vi "runtest Run Single Test.vi"(6 "TestStation IP (\"\")":string, 7 "Fields In":T1[](array[typedef]), 8 "error in (no error)":errorcluster, 9 "Test Execution Settings":T4={"Quick Mode (T)"=FALSE, "Seq Count"=0, "Step Info"="", "Instruments on Station"=[], "LANGUAGE"="English", "Files Found?"=FALSE, "Step Number"=1} {"Step Number" min=1 step=1}, 10 "Test Configuration (\"\")":string, 11 "Test_ID (\"\")":string) -> (0 "error out":errorcluster, 3 "Fields Out":T1[](array[typedef]), 5 "Test Output":T6)   [LabVIEW 2011]
uses:
  tests/Test Output.ctl
  tests/Test Execution Settings.ctl
  server/database/Stations/Instruments/Instrument Record.ctl
  server/database/Fields/Field Record.ctl
  server/database/Fields/Field DataTypes.ctl
  server/database/Fields/Field NextItem.ctl
  server/database/Fields/Field System Fields.ctl
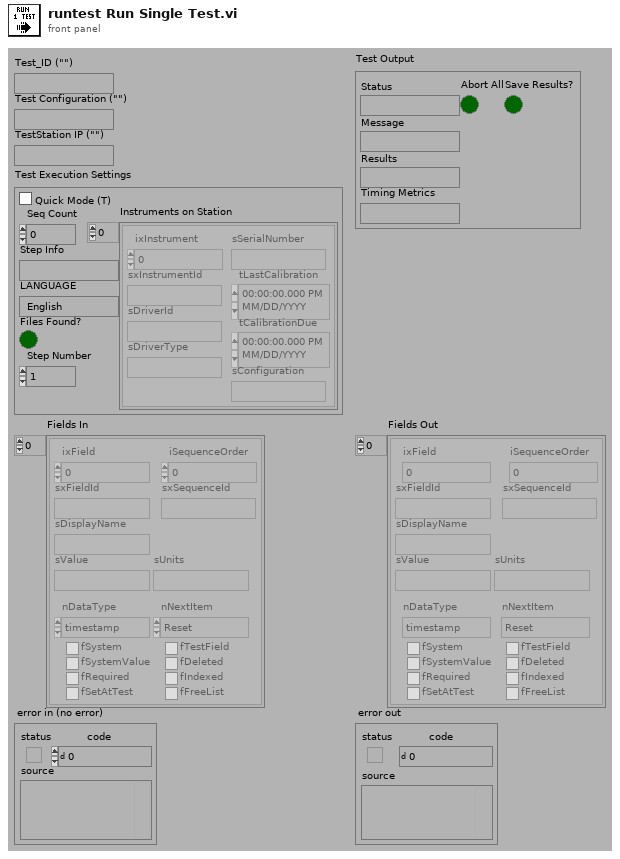
[diagram p1: front panel]
types:
  T1 = typedef "Field Record.ctl" = cluster{"ixField":i32, "iSequenceOrder":i32, "sxFieldId":string, "sxSequenceId":string, "sDisplayName":string, "sValue":string, "sUnits":string, "nDataType":T2, "nNextItem":T3, "fSystem":bool, "fSystemValue":bool, "fRequired":bool, "fSetAtTest":bool, "fTestField":bool, "fDeleted":bool, "fIndexed":bool, "fFreeList":bool}
  T2 = typedef "Field DataTypes.ctl" = enum32{"text", "numeric", "list", "timestamp", "boolean"}
  T3 = typedef "Field NextItem.ctl" = enum32{"Reset", "Retain", "Auto-Increment"}
  T4 = typedef "Test Execution Settings.ctl" = cluster{"Quick Mode (T)":bool, "Seq Count":i32, "Step Info":string, "Instruments on Station":T5[], "LANGUAGE":string, "Files Found?":bool, "Step Number":i32}
  T5 = typedef "Instrument Record.ctl" = cluster{"ixInstrument":i32, "sxInstrumentId":string, "sDriverId":string, "sDriverType":string, "sSerialNumber":string, "tLastCalibration":timestamp, "tCalibrationDue":timestamp, "sConfiguration":string}
  T6 = typedef "Test Output.ctl" = cluster{"Status":string, "Message":string, "Results":string, "Abort All":bool, "Save Results?":bool, "Timing Metrics":string}
  T7 = typedef "Field System Fields.ctl" = enum32{"Company", "End_Timestamp", "Model_Number", "Operator", "Serial_Number", "Start_Timestamp", "Step_Number", "Step_Tag", "Test_Run", "Test_Sequence", "Test_Station", "Test_Station_Name", "Test_Status", "Test_Type", "Test_Version", "Spartan_Version_Created", "Spartan_Version_Current"}
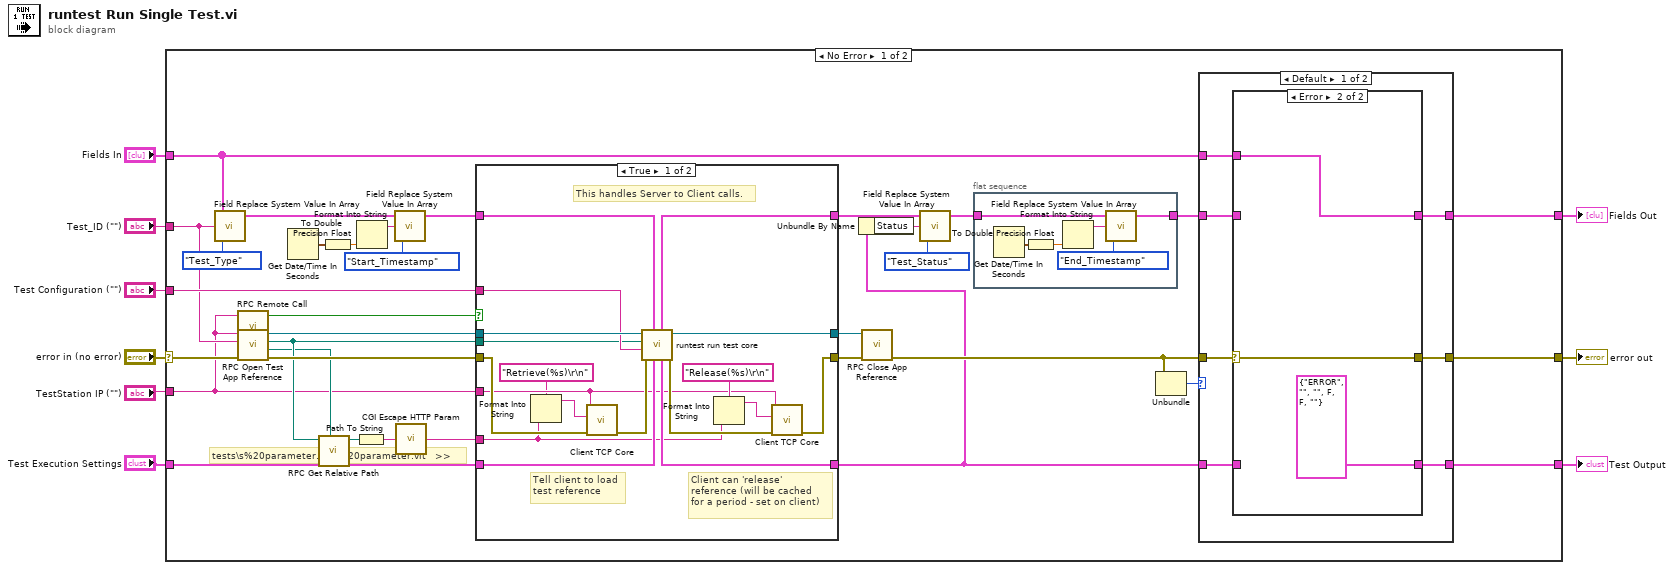
[diagram p0: block diagram]
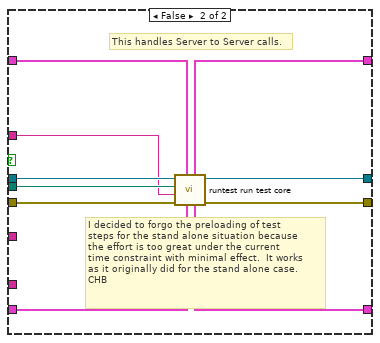
[diagram p2: hidden frame]
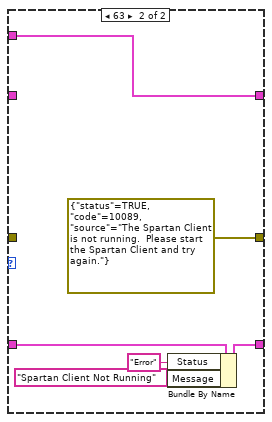
[diagram p4: hidden frame]
diagram:
  n1 = case shown="No Error" "error in (no error)" {
    selector: "error in (no error)" -> [w16 w97]
    tunnel: [w42 _] -> w9
    tunnel: "Test_ID (\"\")" -> [w14 _]
    tunnel: "Test Execution Settings" -> [w39 _]
    tunnel: "Test Configuration (\"\")" -> [w38 _]
    tunnel: [w35 w97] -> w5
    tunnel: [w34 w98] -> w4
    tunnel: "Fields In" -> [w33 w98]
    tunnel: "TestStation IP (\"\")" -> [w11 _]
    frame No Error {
      # "tests\\s%20parameter.dll\\s%20parameter.vit   >>"
      n2 = call "Field Replace System Value In Array.vi"("System Field to Replace (Serial Number)"=Field_System_Fields."Test_Type", "Field Value Replacement Data (\"\")"=w14, "Fields Array In"=w33) -> ("Fields Array Out"=w30:T1[])  [unwired: 1 in, 1 out]
      n3 = call "RPC Remote Call.vi"("IP (\"\")"=w11) -> ("Remote Call?"=w10:bool)  [unwired: 4 out]
      n4 = call "RPC Open Test App Reference.vi"("error in (no error)"=w16, "Test ID (\"\")"=w14, "Client (\"\": open server reference)"=w11) -> ("error out"=w17:errorcluster, "Component Base Path"=w12:path, "Test Component Path"=w13:path, "app reference"=w15:refnum<vi>)  [unwired: 1 in, 4 out]
      n5 = Get Date/Time In Seconds() -> (seconds since 1Jan1904=w28:timestamp)
      n6 = call "RPC Get Relative Path.vi"("Base Path (empty)"=w12, "Absolute Path (empty)"=w13) -> ("Path Relative to Base"=w20:path)  [unwired: 3 out]
      n7 = To Double Precision Float(number=w28) -> (double precision float=w27:dbl)
      n8 = Path To String(path=w20) -> (string=w19:string)
      n9 = Format Into String(w27) -> (resulting string=w31:string)  [unwired: 3 in, 1 out]
      n10 = call "Field Replace System Value In Array.vi"("System Field to Replace (Serial Number)"=Field_System_Fields."Start_Timestamp", "Field Value Replacement Data (\"\")"=w31, "Fields Array In"=w30) -> ("Fields Array Out"=w29:T1[])  [unwired: 1 in, 1 out]
      n11 = call "CGI Escape HTTP Param.vi"("string"=w19) -> ("url-encoded string"=w18:string)
      n12 = case shown="True" w10 {
        tunnel: w15 -> [w64 w76]
        tunnel: w29 -> [w67 w77]
        tunnel: w39 -> [w63 w70]
        tunnel: w38 -> [w61 w71]
        tunnel: [w66 w74] -> w37
        tunnel: [w62 w68] -> w21
        tunnel: w17 -> [w60 w72]
        tunnel: [w57 w69] -> w26
        tunnel: [w65 w75] -> w36
        tunnel: w13 -> [w51 w73]
        tunnel: w11 -> [w55 _]
        tunnel: w18 -> [w50 _]
        frame True {
          # "Client can 'release'\nreference (will be cached\nfor a period - set on client)"
          # "Tell client to load\ntest reference"
          # "This handles Server to Client calls."
          n13 = Format Into String(format string="Retrieve(%s)\r\n" ("Command(Params) (\"\")"), w50) -> (resulting string=w52:string)  [unwired: 2 in, 1 out]
          n14 = call "Client TCP Core.vi"("error in (no error)"=w60, "Command(Params) (\"\")"=w52, "Client (\"\": localhost)"=w55) -> ("error out"=w59:errorcluster)  [unwired: 8 out]
          n15 = call "runtest run test core.vi"("Test Execution Settings"=w63, "Fields In"=w67, "error in (no error)"=w59, "Parameters"=w61, "Test Path (empty)"=w51, "application reference (local)"=w64) -> ("error out"=w58:errorcluster, "dup application reference"=w65:refnum<vi>, "Test Output"=w62:T6, "Fields Out"=w66:T1[])  [unwired: 2 out]
          n16 = Format Into String(format string="Release(%s)\r\n" ("Command(Params) (\"\")"), w50) -> (resulting string=w54:string)  [unwired: 2 in, 1 out]
          n17 = call "Client TCP Core.vi"("error in (no error)"=w58, "Command(Params) (\"\")"=w54, "Client (\"\": localhost)"=w55) -> ("error out"=w57:errorcluster)  [unwired: 8 out]
        }
        frame False {
          # "I decided to forgo the preloading of test\nsteps for the stand alone situation because\nthe effort is too great under the current\ntime constraint with minimal effect.  It works\nas it originally did for the stand alone case.\nCHB"
          # "This handles Server to Server calls."
          n18 = call "runtest run test core.vi"("Test Execution Settings"=w70, "Fields In"=w77, "error in (no error)"=w72, "Parameters"=w71, "Test Path (empty)"=w73, "application reference (local)"=w76) -> ("error out"=w69:errorcluster, "dup application reference"=w75:refnum<vi>, "Test Output"=w68:T6, "Fields Out"=w74:T1[])  [unwired: 2 out]
        }
      }
      n19 = Unbundle By Name(w21) -> ("Status"=w24:string)
      n20 = call "RPC Close App Reference.vi"("error in (no error)"=w26, "app reference"=w36) -> ("error out"=w25:errorcluster)  [unwired: 9 out]
      n21 = call "Field Replace System Value In Array.vi"("System Field to Replace (Serial Number)"=Field_System_Fields."Test_Status", "Field Value Replacement Data (\"\")"=w24, "Fields Array In"=w37) -> ("Fields Array Out"=w23:T1[])  [unwired: 1 in, 1 out]
      n22 = flat-sequence {
        tunnel: w23 -> [w46]
        tunnel: [w45] -> w22
        frame #0 {
          n23 = Get Date/Time In Seconds() -> (seconds since 1Jan1904=w49:timestamp)
          n24 = To Double Precision Float(number=w49) -> (double precision float=w48:dbl)
          n25 = Format Into String(w48) -> (resulting string=w44:string)  [unwired: 3 in, 1 out]
          n26 = call "Field Replace System Value In Array.vi"("System Field to Replace (Serial Number)"=Field_System_Fields."End_Timestamp", "Field Value Replacement Data (\"\")"=w44, "Fields Array In"=w46) -> ("Fields Array Out"=w45:T1[])  [unwired: 1 in, 1 out]
        }
      }
      n27 = Unbundle(w25) -> ("code"=w43:i32)  [unwired: 2 out]
      n28 = case shown="Default" w43 {
        tunnel: w21 -> [w78 w96]
        tunnel: [w79 w95] -> w42
        tunnel: w25 -> [w84 _]
        tunnel: [w80 errorcluster {"status"=TRUE, "code"=10089, "source"="The Spartan Client is not running.  Please start the Spartan Client and try again."} ("error out")] -> w35
        tunnel: w33 -> [w81 w91]
        tunnel: w22 -> [w83 _]
        tunnel: [w82 w91] -> w34
        frame Default {
          n29 = case shown="Error" w84 {
            selector: w84 -> [w85 w89]
            tunnel: w83 -> [w87 _]
            tunnel: [w87 w90] -> w82
            tunnel: w81 -> [_ w90]
            tunnel: [w85 w89] -> w80
            tunnel: [w86 T6 {"Status"="ERROR", "Message"="", "Results"="", "Abort All"=FALSE, "Save Results?"=FALSE, "Timing Metrics"=""} ("Test Output")] -> w79
            tunnel: w78 -> [w86 _]
            frame No Error {
            }
            frame Error {
            }
          }
        }
        frame 63 {
          n30 = Bundle By Name(cluster=w96, "Status"="Error", "Message"="Spartan Client Not Running" ("Status")) -> (w95:T6)
        }
      }
    }
    frame Error {
    }
  }
  "error out" <- w5
  "Test Output" <- w9
  "Fields Out" <- w4
